vi "niDTS DUT to WLAN DUT.vi"(9 "error in":errorcluster, 10 "Dut Handle":T2) -> (1 "error out":errorcluster, 2 "WLAN Dut Handle":T1)   [LabVIEW 2015, in "niDTS WLAN.lvlib" / "niDTS WLAN Dut.lvclass"]
uses:
  niDTS WLAN Dut.lvclass
  Framework/Dut/Includes/niDTS Dut INC Handle.ctl
  Framework/Dut/Objects/BASE_class/niDTS Dut.lvclass
  Includes/niDTS WLAN Dut INC Handle.ctl
  niDTS WLAN.lvlib
  Framework/niDTS Framework.lvlib
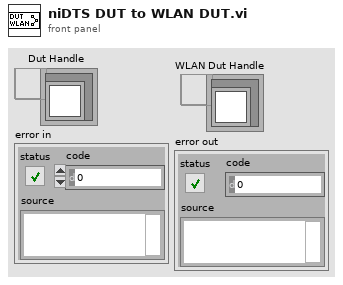
[diagram p1: front panel]
types:
  T1 = typedef "niDTS WLAN.lvlib/niDTS WLAN Dut INC Handle.ctl" = refnum<data-value>
  T2 = typedef "niDTS Framework.lvlib/niDTS Dut INC Handle.ctl" = refnum<data-value>
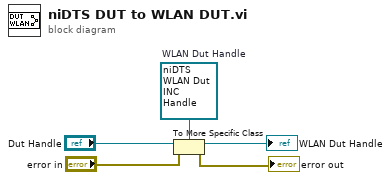
[diagram p0: block diagram]
diagram:
  w5 = T1 refnum  # WLAN Dut Handle
  n1 = To More Specific Class(target class=w5, reference="Dut Handle", error in="error in") -> (specific class reference=→"WLAN Dut Handle":T1, error out=→"error out":errorcluster)
